vi "UIRef.vi"(8 "error in":errorcluster, 11 "node in":refnum<class "VI modification collection.lvclass">) -> (0 "error out":errorcluster, 2 "VI refnum":refnum<vi>, 3 "node out":refnum<class "VI modification collection.lvclass">)   [LabVIEW 2013, in "VI modification collection.lvclass"]
doc: "Stores the static reference to the UI of the node."
uses:
  VI modification collection.lvclass
  execution ui.vi
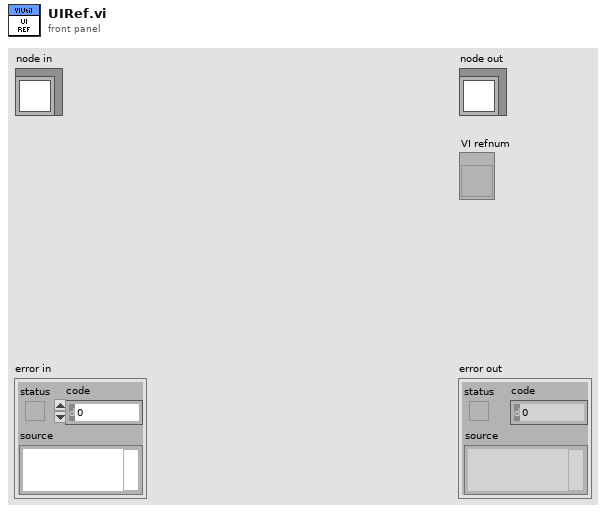
[diagram p1: front panel]
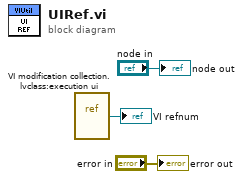
[diagram p0: block diagram]
diagram:
  n1 = vi-ref "VI modification collection.lvclass:execution ui.vi"() -> (→"VI refnum":refnum<vi>)
  "error out" <- "error in"
  "node out" <- "node in"
